vi "read buffer Date.vi"(8 "error in (no error)":errorcluster caption="错误输入（无错误）", 11 "串口参数管理 输入":refnum<class "串口通讯.lvclass">) -> (0 "error out":errorcluster caption="错误输出", 2 "读取缓冲区":string, 3 "串口参数管理 输出":refnum<class "串口通讯.lvclass">)   [LabVIEW 2015, in "串口通讯.lvlib" / "串口通讯.lvclass"]
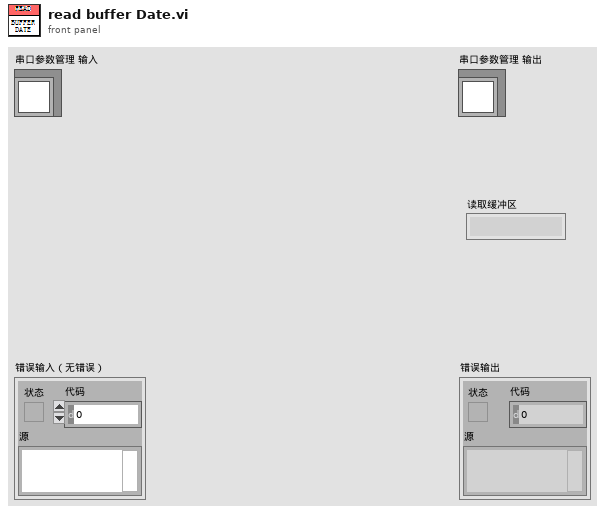
[diagram p1: front panel]
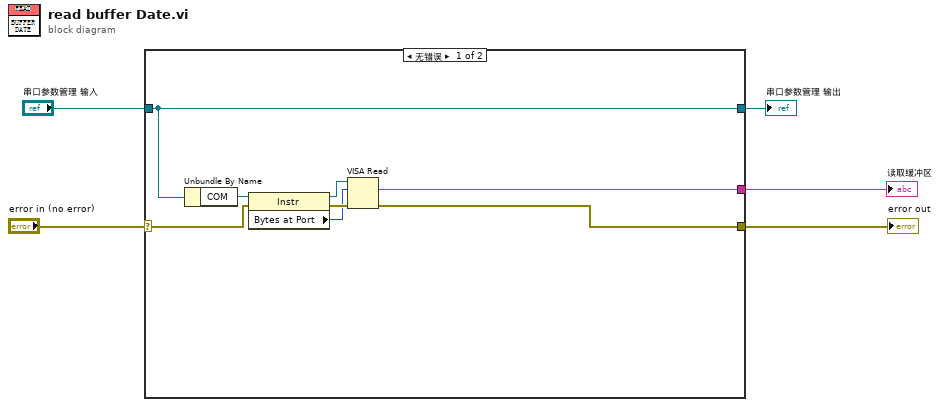
[diagram p0: block diagram]
diagram:
  n1 = case shown="无错误" "error in (no error)" {
    selector: "error in (no error)" -> [w8 w15]
    tunnel: [w9 w15] -> w4
    tunnel: [w7 w14] -> w2
    tunnel: "串口参数管理 输入" -> [w7 w14]
    tunnel: [w6 _] -> w1
    frame No Error {
      n2 = Unbundle By Name(w7) -> ("COM"=w13:refnum<visa-resource-name>)
      n3 = property class="Instr"(reference=w13, error in=w8) -> (reference out=w12:refnum<visa-resource-name>, error out=w11:errorcluster, "Bytes at Port"=w10:u32)
      n4 = VISA Read(VISA resource name=w12, byte count=w10, error in (no error)=w11) -> (read buffer=w6:string, error out=w9:errorcluster)  [unwired: 2 out]
    }
    frame Error {
    }
  }
  "error out" <- w4
  "串口参数管理 输出" <- w2
  "读取缓冲区" <- w1
